vi "prueba lcd.vi"() -> ()   [LabVIEW 2013]
uses:
  <vilib>/LabVIEW Interface for Arduino/Type Defs/LCD Pin Config 4 bit.ctl
  <vilib>/LabVIEW Interface for Arduino/Type Defs/Arduino Resource.ctl
  <vilib>/LabVIEW Interface for Arduino/Type Defs/Board Type.ctl
  <vilib>/LabVIEW Interface for Arduino/Type Defs/Pin Mode.ctl
  <vilib>/LabVIEW Interface for Arduino/Type Defs/Direction.ctl
  <vilib>/Utility/file.llb/Write To Spreadsheet File (string).vi
  <vilib>/LabVIEW Interface for Arduino/LabVIEW Interface for Arduino.lvlib
panel:
  in  "LCD Pin Config 4 Bit 2":T1={"RS"=12, "RW"=255, "Enable"=11, "D4"=5, "D5"=4, "D6"=3, "D7"=2, "LCD"=10}
  out "output variable":dbl
  out "Arduino Resource 2":T2={"VISA resource"="", "Board Type"=enum."Uno", "Connection Type"=enum."USB / Serial", "Bytes Per Packet (15)"=15}
  out "error out 2":errorcluster
  in  "LCD Pin Config 4 Bit":T1={"RS"=12, "RW"=255, "Enable"=11, "D4"=5, "D5"=4, "D6"=3, "D7"=2, "LCD"=10}
  in  "stop":bool
  out "x*y":u8
  out "Voltage":dbl(knob) scale=0.0..5.0
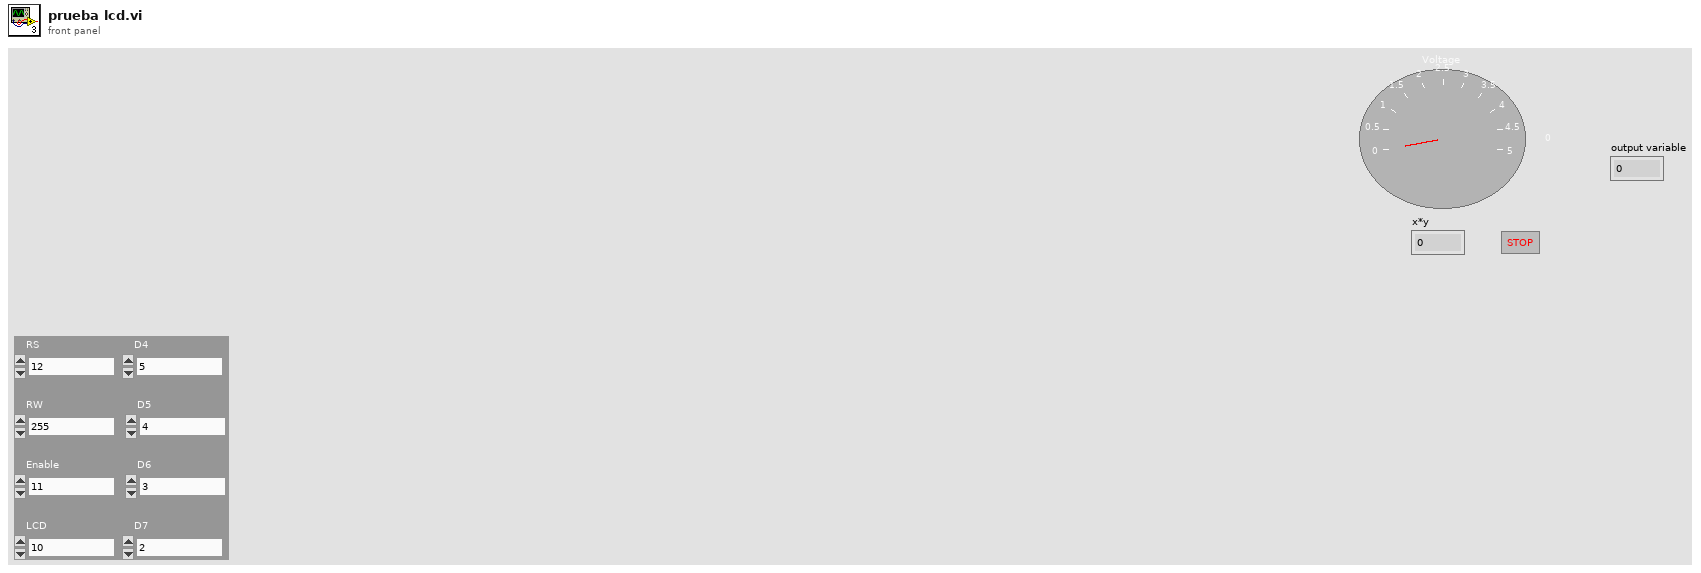
[diagram p1: front panel]
types:
  T1 = typedef "LabVIEW Interface for Arduino.lvlib/LCD Pin Config 4 bit.ctl" = cluster{"RS":u8, "RW":u8, "Enable":u8, "D4":u8, "D5":u8, "D6":u8, "D7":u8, "LCD":u8}
  T2 = typedef "LabVIEW Interface for Arduino.lvlib/Arduino Resource.ctl" = cluster{"VISA resource":refnum<visa-resource-name>, "Board Type":T3, "Connection Type":enum8{"USB / Serial"}, "Bytes Per Packet (15)":u8}
  T3 = typedef "LabVIEW Interface for Arduino.lvlib/Board Type.ctl" = enum16{"Uno", "Dimuelanove w/Atmega 328", "Mega 2560"}
  T4 = typedef "LabVIEW Interface for Arduino.lvlib/Direction.ctl" = enum8{"Left ", "Right"}
  T5 = typedef "LabVIEW Interface for Arduino.lvlib/Pin Mode.ctl" = enum8{"Input", "Output"}
  T6 = enum8{"String", "Binary", "Decimal", "Octal", "Hexadecimal"}
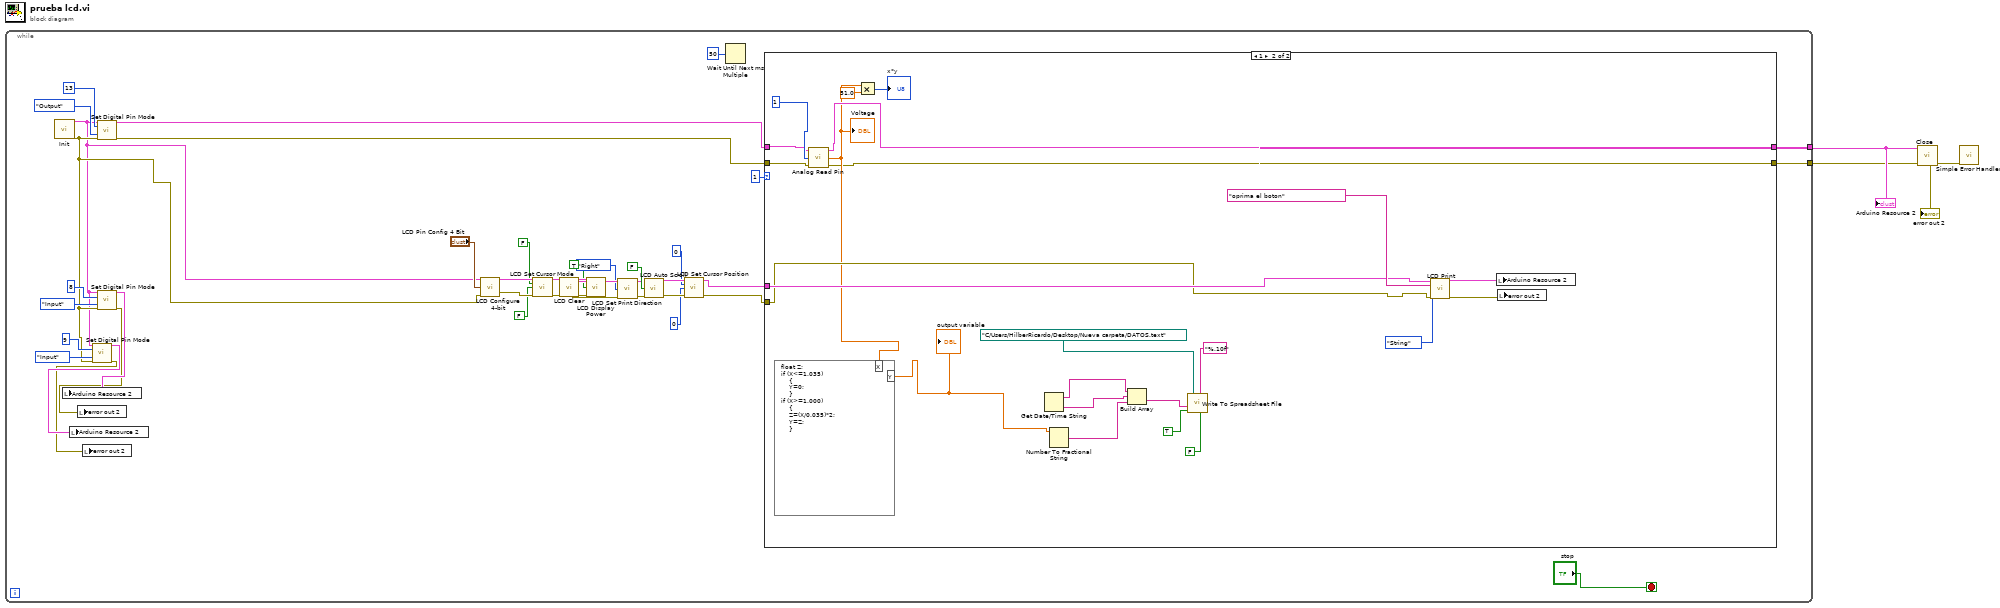
[diagram p0: block diagram]
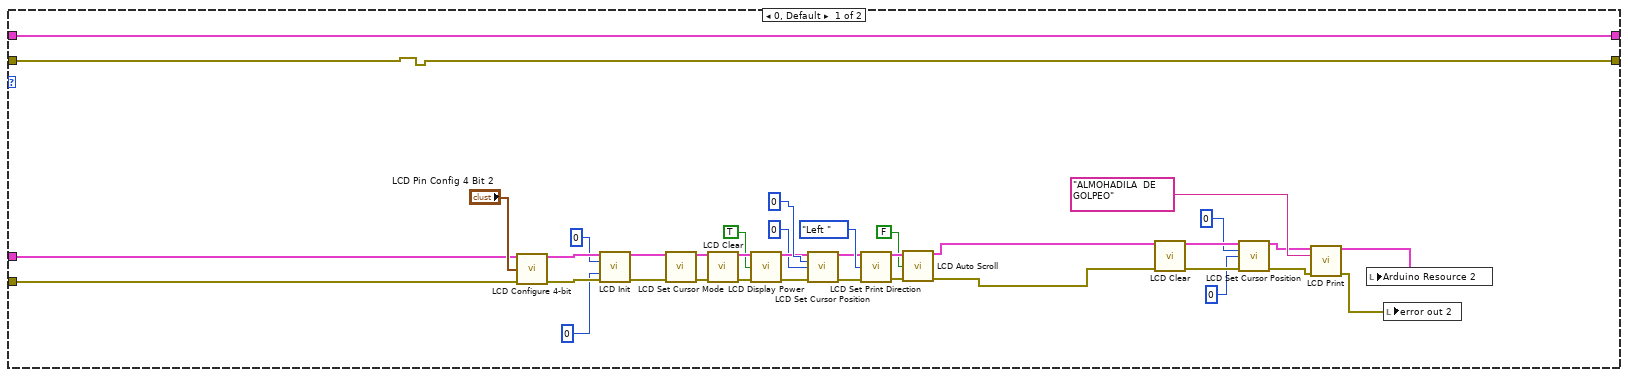
[diagram p2: hidden frame]
diagram:
  n1 = while {
    tunnel: [w44] -> w3
    tunnel: [w43] -> w2
    stop <- "stop" stop-if-true
    n2 = call <vilib>:"Init.vi"() -> ("Arduino Resource"=w11:T2, "error out"=w12:errorcluster)  [unwired: 18 in]
    n3 = call <vilib>:"Set Digital Pin Mode.vi"("Arduino Resource"=w11, "Digital I/O Pin"=u8 9, "Pin Mode (Input)"=Pin_Mode."Input", "error in"=w12) -> ("Arduino Resource"=w40:T2, "error out"=w38:errorcluster)  [unwired: 10 in]
    n4 = local write "Arduino Resource 2"(w40) -> ()
    n5 = local write "error out 2"(w38) -> ()
    n6 = call <vilib>:"Set Digital Pin Mode.vi"("Arduino Resource"=w11, "Digital I/O Pin"=u8 13, "Pin Mode (Input)"=Pin_Mode."Output", "error in"=w12) -> ("Arduino Resource"=w30:T2, "error out"=w29:errorcluster)  [unwired: 10 in]
    n7 = call <vilib>:"Set Digital Pin Mode.vi"("Arduino Resource"=w11, "Digital I/O Pin"=u8 8, "Pin Mode (Input)"=Pin_Mode."Input", "error in"=w12) -> ("Arduino Resource"=w39:T2, "error out"=w37:errorcluster)  [unwired: 10 in]
    n8 = local write "Arduino Resource 2"(w39) -> ()
    n9 = local write "error out 2"(w37) -> ()
    n10 = call <vilib>:"LCD Configure 4-bit.vi"("Arduino Resource"=w11, "LCD Pin Config 4 Bit"="LCD Pin Config 4 Bit", "error in"=w12) -> ("Arduino Resource"=w27:T2, "error out"=w28:errorcluster)  [unwired: 11 in]
    n11 = call <vilib>:"LCD Set Cursor Mode.vi"("Arduino Resource"=w27, "Cursor On? (T)"=FALSE, "Cursor Blink? (F)"=FALSE, "error out"=w28) -> ("Arduino Resource"=w18:T2, "error out"=w17:errorcluster)  [unwired: 10 in]
    n12 = call <vilib>:"LCD Clear.vi"("Arduino Resource"=w18, "error in"=w17) -> ("Arduino Resource"=w19:T2, "error out"=w20:errorcluster)  [unwired: 12 in]
    n13 = call <vilib>:"LCD Display Power.vi"("Arduino Resource"=w19, "Display On? (T) 2"=TRUE, "error in"=w20) -> ("Arduino Resource"=w23:T2, "error out"=w24:errorcluster)  [unwired: 11 in]
    n14 = call <vilib>:"LCD Set Print Direction.vi"("Arduino Resource"=w23, "Print Direction"=Direction."Right" ("Direction"), "error in"=w24) -> ("Arduino Resource"=w14:T2, "error"=w13:errorcluster)  [unwired: 11 in]
    n15 = call <vilib>:"LCD Auto Scroll.vi"("Arduino Resource"=w14, "Auto Scroll?"=FALSE ("Auto Scroll? 2"), "error in"=w13) -> ("Arduino Resource"=w10:T2, "error out"=w9:errorcluster)  [unwired: 11 in]
    n16 = call <vilib>:"LCD Set Cursor Position.vi"("Arduino Resource"=w10, "Column"=u8 0, "Row"=u8 0, "error out"=w9) -> ("Arduino Resource"=w6:T2, "error out"=w5:errorcluster)  [unwired: 10 in]
    n17 = Wait Until Next ms Multiple(millisecond multiple=u32 50) -> ()  [unwired: 1 out]
    n18 = case shown="1" u8 1 {
      tunnel: w29 -> [w73 w84]
      tunnel: w30 -> [w74 w82]
      tunnel: [w74 w87] -> w44
      tunnel: [w73 w85] -> w43
      tunnel: w6 -> [w46 w89]
      tunnel: w5 -> [w45 w88]
      frame 0, Default {
        n19 = call <vilib>:"LCD Configure 4-bit.vi"("Arduino Resource"=w46, "LCD Pin Config 4 Bit"="LCD Pin Config 4 Bit 2", "error in"=w45) -> ("Arduino Resource"=w51:T2, "error out"=w52:errorcluster)  [unwired: 11 in]
        n20 = call <vilib>:"LCD Init.vi"("Arduino Resource"=w51, "Columns"=u8 0, "Rows"=u8 0, "error in"=w52) -> ("Arduino Resource"=w66:T2, "error out"=w67:errorcluster)  [unwired: 10 in]
        n21 = call <vilib>:"LCD Set Cursor Mode.vi"("Arduino Resource"=w66, "error out"=w67) -> ("Arduino Resource"=w60:T2, "error out"=w61:errorcluster)  [unwired: 12 in]
        n22 = call <vilib>:"LCD Clear.vi"("Arduino Resource"=w60, "error in"=w61) -> ("Arduino Resource"=w59:T2, "error out"=w58:errorcluster)  [unwired: 12 in]
        n23 = call <vilib>:"LCD Display Power.vi"("Arduino Resource"=w59, "Display On? (T) 2"=TRUE, "error in"=w58) -> ("Arduino Resource"=w56:T2, "error out"=w55:errorcluster)  [unwired: 11 in]
        n24 = call <vilib>:"LCD Set Cursor Position.vi"("Arduino Resource"=w56, "Column"=u8 0, "Row"=u8 0, "error out"=w55) -> ("Arduino Resource"=w63:T2, "error out"=w64:errorcluster)  [unwired: 10 in]
        n25 = call <vilib>:"LCD Set Print Direction.vi"("Arduino Resource"=w63, "Print Direction"=Direction."Left " ("Direction"), "error in"=w64) -> ("Arduino Resource"=w69:T2, "error"=w70:errorcluster)  [unwired: 11 in]
        n26 = call <vilib>:"LCD Auto Scroll.vi"("Arduino Resource"=w69, "Auto Scroll?"=FALSE ("Auto Scroll? 2"), "error in"=w70) -> ("Arduino Resource"=w48:T2, "error out"=w47:errorcluster)  [unwired: 11 in]
        n27 = call <vilib>:"LCD Clear.vi"("Arduino Resource"=w48, "error in"=w47) -> ("Arduino Resource"=w77:T2, "error out"=w78:errorcluster)  [unwired: 12 in]
        n28 = call <vilib>:"LCD Set Cursor Position.vi"("Arduino Resource"=w77, "Column"=u8 0, "Row"=u8 0, "error out"=w78) -> ("Arduino Resource"=w79:T2, "error out"=w80:errorcluster)  [unwired: 10 in]
        n29 = call <vilib>:"LCD Print.vi"("Arduino Resource"=w79, "Data"="ALMOHADILA  DE GOLPEO", "error out"=w80) -> ("Arduino Resource"=w72:T2, "error out"=w71:errorcluster)  [unwired: 11 in]
        n30 = local write "Arduino Resource 2"(w72) -> ()
        n31 = local write "error out 2"(w71) -> ()
      }
      frame 1 {
        n32 = call <vilib>:"Analog Read Pin.vi"("Arduino Resource"=w82, "Analog Input Pin (0)"=u8 1, "error in"=w84) -> ("Arduino Resource"=w87:T2, "Voltage"=w86:dbl, "error out"=w85:errorcluster)  [unwired: 10 in]
        "Voltage" <- w86
        n33 = formula code="float Z;\nif (X<=1.035)\n    {\n    Y=0;\n    }\nif (X>=1.000)\n    {\n    Z=(X/0.035)*2;\n    Y=Z;\n    }"("X"=w86) -> ("Y"=w92:dbl)
        "output variable" <- w92
        n34 = Multiply(x=w86, y=51.0) -> (x*y=→"x*y":u8)
        n35 = Get Date/Time String() -> (date string=w97:string, time string=w96:string)  [unwired: 3 in]
        n36 = Number To Fractional String(number=w92) -> (F-format string=w95:string)  [unwired: 3 in]
        n37 = Build Array(w97, w96, w95) -> (w100:string[])
        n38 = call-poly <vilib>:"Write To Spreadsheet File.vi"("transpose? (no:F)"=FALSE, "format (%s)"="%.10f" ("format (%.3f)"), "append to file? (new file:F)"=TRUE, "1D data"=w100, "file path (dialog if empty)"=path "C:/Users/HilberRicardo/Desktop/Nueva carpeta/DATOS.text") -> ()  [unwired: 3 in, 1 out]
        n39 = call <vilib>:"LCD Print.vi"("Arduino Resource"=w89, "Data"="oprima el boton", "Base (String)"=T6."String", "error out"=w88) -> ("Arduino Resource"=w94:T2, "error out"=w93:errorcluster)  [unwired: 10 in]
        n40 = local write "Arduino Resource 2"(w94) -> ()
        n41 = local write "error out 2"(w93) -> ()
      }
    }
  }
  "error out 2" <- w2
  "Arduino Resource 2" <- w3
  n42 = call <vilib>:"Close.vi"("Arduino Resource"=w3, "error in"=w2) -> ("error out"=w1:errorcluster)  [unwired: 13 in]
  n43 = call <vilib>:"Simple Error Handler.vi"("error in (no error)"=w1) -> ()  [unwired: 4 in, 5 out]
